vi "更新102站.vi"() -> ()   [LabVIEW 2014]
uses:
  <vilib>/addons/database/Connection.llb/DB Tools Open Connec (String).vi
  <vilib>/addons/database/NI_Database_API.lvlib
panel:
  in  "QRcode":string
  in  "更新10-错位__单个":bool
  out "数据":string[][](array[string])
  in  "路径":path
  in  "读取文件表格":bool
  in  "更新10-错位__批量":bool
  in  "停止":bool
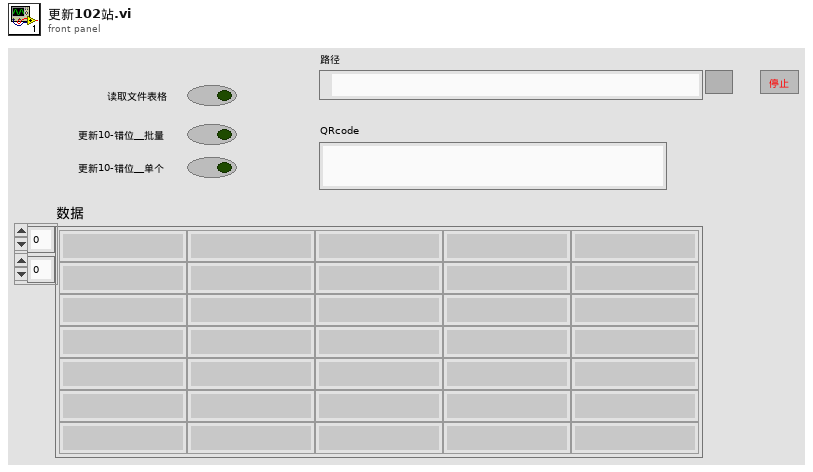
[diagram p1: front panel]
types:
  T1 = typedef "NI_Database_API.lvlib/Conn ObjectReference.ctl" = refnum<k1>
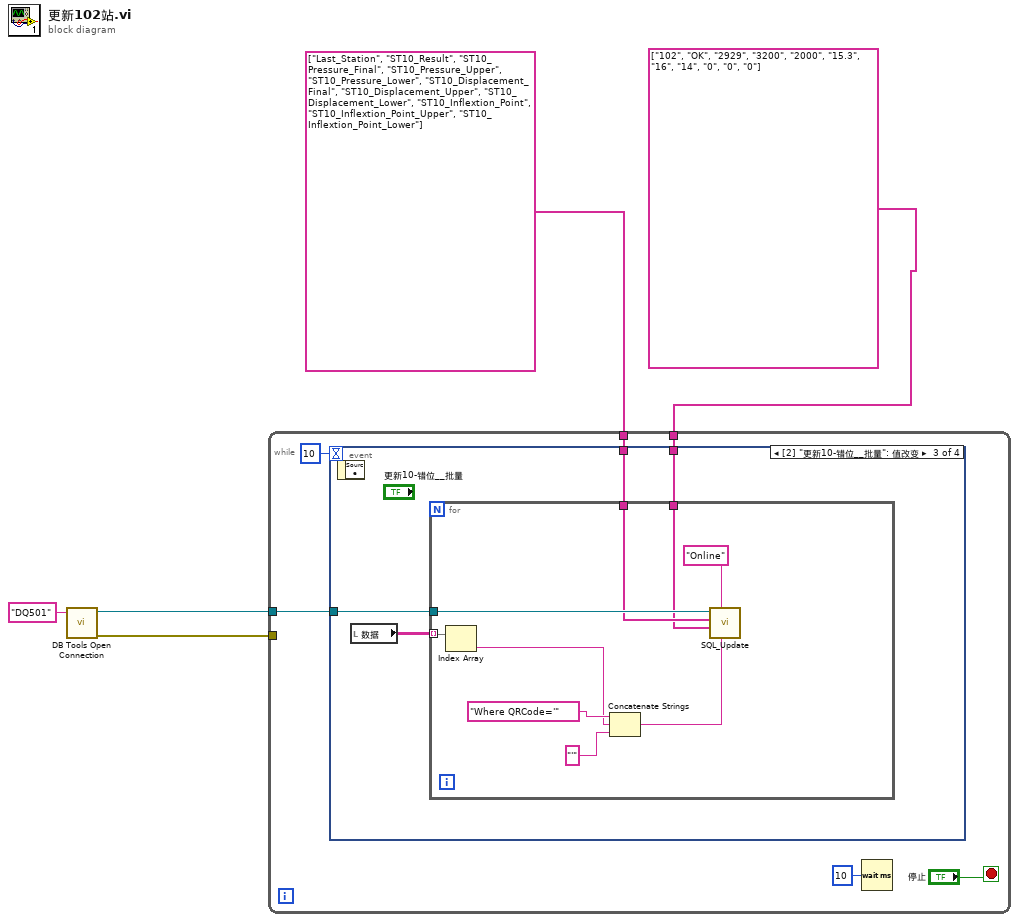
[diagram p0: block diagram]
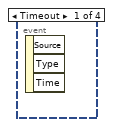
[diagram p2: hidden frame]
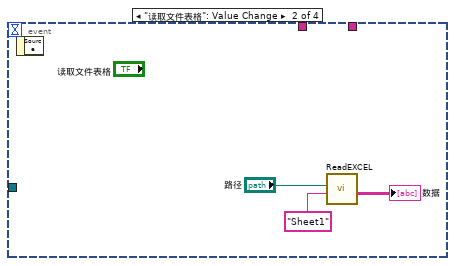
[diagram p3: hidden frame]
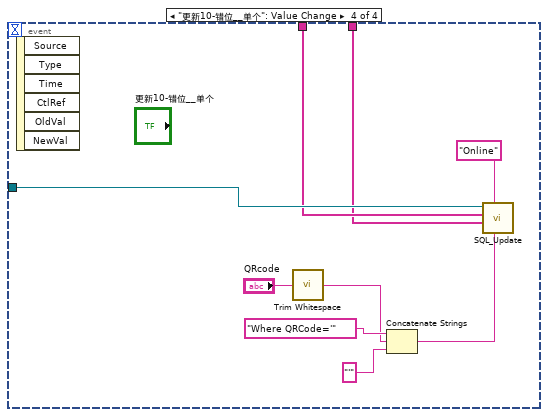
[diagram p4: hidden frame]
diagram:
  n1 = call-poly <vilib>:"DB Tools Open Connection.vi"("connection information"="DQ501") -> ("error out"=w3:errorcluster, "connection reference"=w4:T1)  [unwired: 7 in]
  n2 = while {
    tunnel: w4 -> [w8]
    tunnel: w3 -> [_]
    tunnel: string[] ["Last_Station", "ST10_Result", "ST10_Pressure_Final", "ST10_Pressure_Upper", "ST10_Pressure_Lower", "ST10_Displacement_Final", "ST10_Displacement_Upper", "ST10_Displacement_Lower", "ST10_Inflextion_Point", "ST10_Inflextion_Point_Upper", "ST10_Inflextion_Point_Lower"] -> [w7]
    tunnel: string[] ["102", "OK", "2929", "3200", "2000", "15.3", "16", "14", "0", "0", "0"] -> [w6]
    stop <- "停止" stop-if-true
    n3 = event shown="[2] \"更新10-错位__批量\": 值改变" {
      selector: _ -> [_ _ _ _]
      dyn-events: _ -> [_ _ _ _]
      timeout: 10 -> [_ _ _ _]
      tunnel: w8 -> [_ _ w17 w32]
      tunnel: w7 -> [_ _ w16 w31]
      tunnel: w6 -> [_ _ w15 w30]
      event Timeout {
        n4 = event-data() -> ()  [unwired: 1 in, 3 out]
      }
      event "读取文件表格": Value Change {
        n5 = event-data() -> ()  [unwired: 1 in, 1 out]
        n6 = call "ReadEXCEL.vi"("EXCEL 标签"="Sheet1", "路径"="路径") -> ("数据"=→"数据":string[][])  [unwired: 8 in, 1 out]
      }
      event "更新10-错位__批量": Value Change {
        n7 = event-data() -> ()  [unwired: 1 in, 1 out]
        n8 = local read "数据"() -> (w18:string[][])
        n9 = for {
          tunnel: w18 -> [w24] mode=indexing
          tunnel: w17 -> [w21]
          tunnel: w16 -> [w20]
          tunnel: w15 -> [w19]
          n10 = Index Array(array=w24) -> (element=w23:string)  [unwired: 1 in]
          n11 = Concatenate Strings("Where QRCode='" ("查询语句"), w23, "'" ("字符串")) -> (w22:string)
          n12 = call "SQL_Update.vi"("查询语句"=w22, "表名"="Online", "列名对应的值"=w19, "列名"=w20, "connection reference"=w21) -> ()  [unwired: 5 in, 2 out]
        }
      }
      event "更新10-错位__单个": Value Change {
        n13 = event-data() -> ()  [unwired: 1 in, 6 out]
        n14 = call <vilib>:"Trim Whitespace.vi"("string"="QRcode") -> ("trimmed string"=w28:string)  [unwired: 1 in]
        n15 = Concatenate Strings("Where QRCode='" ("查询语句"), w28, "'" ("字符串")) -> (w33:string)
        n16 = call "SQL_Update.vi"("查询语句"=w33, "表名"="Online", "列名对应的值"=w30, "列名"=w31, "connection reference"=w32) -> ()  [unwired: 5 in, 2 out]
      }
    }
    n17 = Wait (ms)(milliseconds to wait=u32 10 ("等待时间（毫秒）")) -> ()  [unwired: 1 out]
  }
